vi "Copy System Data.vi"(8 "error in (no error)":errorcluster, 10 "System Original":refnum<class "System.lvclass">, 11 "System in":refnum<class "System.lvclass">) -> (0 "error out":errorcluster, 3 "System out":refnum<class "System.lvclass">)   [LabVIEW 2013, in "System.lvclass"]
uses:
  System.lvclass
  System.lvclass/System.ctl
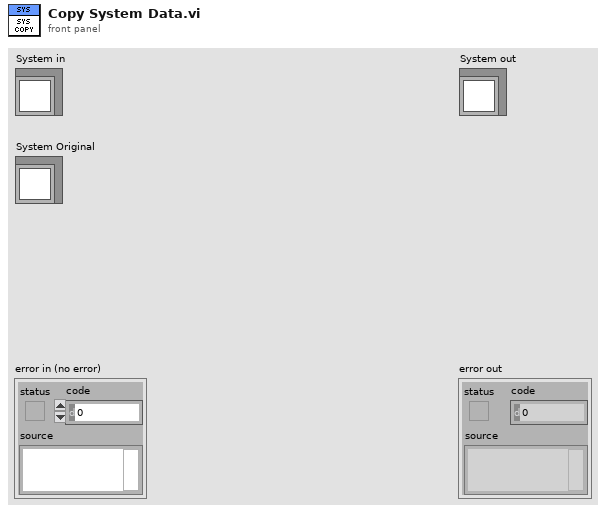
[diagram p1: front panel]
types:
  T1 = cluster{"Has Begun":bool, "Is Running":bool, "Has Finished":bool}
  T2 = typedef "Semaphore RefNum" = refnum<k1>
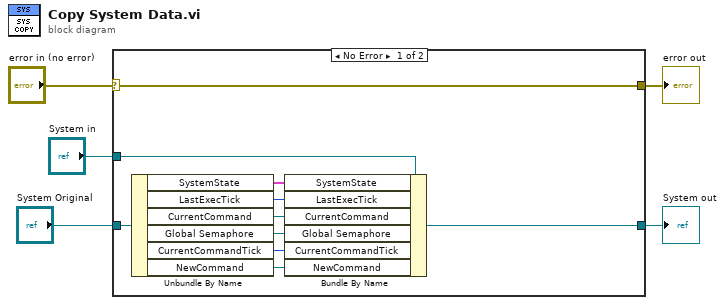
[diagram p0: block diagram]
diagram:
  n1 = case shown="No Error" "error in (no error)" {
    selector: "error in (no error)" -> [w14 w17]
    tunnel: [w14 w17] -> w4
    tunnel: [w13 w16] -> w2
    tunnel: "System in" -> [w15 w16]
    tunnel: "System Original" -> [w12 _]
    frame No Error {
      n2 = Unbundle By Name(w12) -> ("SystemState"=w11:T1, "LastExecTick"=w10:u32, "CurrentCommand"=w9:refnum<class "Command.lvclass">, "Global Semaphore"=w8:T2, "CurrentCommandTick"=w7:u32, "NewCommand"=w6:refnum<class "Command.lvclass">)
      n3 = Bundle By Name(cluster=w15, "SystemState"=w11, "LastExecTick"=w10, "CurrentCommand"=w9, "Global Semaphore"=w8, "CurrentCommandTick"=w7, "NewCommand"=w6) -> (w13:refnum<class "System.lvclass">)
    }
    frame Error {
    }
  }
  "error out" <- w4
  "System out" <- w2
